vi "Get App Data Dir(冲突时的文件备份2013-03-27 14-08-21).vi"(8 "错误输入":errorcluster) -> (0 "错误输出":errorcluster, 3 "App Data":path)   [LabVIEW 2012, in "Application.lvlib"]
uses:
  Application.lvlib
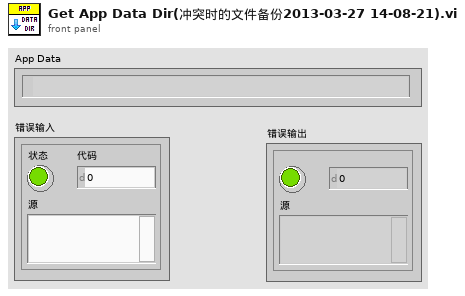
[diagram p1: front panel]
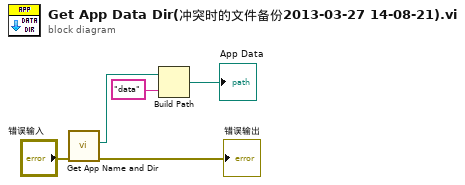
[diagram p0: block diagram]
diagram:
  n1 = call "Get App Name and Dir.vi"("错误输入"="错误输入") -> ("错误输出"=→"错误输出":errorcluster, "AppDir"=w5:path)  [unwired: 8 in, 1 out]
  n2 = Build Path(base path=w5, name or relative path="data" ("名称或相对路径")) -> (appended path=→"App Data":path)
